vi "Sort Fcurve segment metadata.vi"(0 "reference in":refnum<class "metadata.lvclass">, 5 "error in (no error)":errorcluster) -> (14 "reference out":refnum<class "metadata.lvclass">, 19 "error out":errorcluster)   [LabVIEW 2019, in "metadata.lvclass"]
uses:
  metadata.lvclass
  Fcurve segment.ctl
  Segment type--combobox.ctl
panel:
  out "Array 3":string[][](array[string])
  out "Array":dbl[][](array[numeric])
  out "Array 2":string[][](array[string])
  out "Fcurve segment":T1[](array[typedef])
  out "Fcurve segments":i32[][](array[numeric])
  out "number_segments":i32
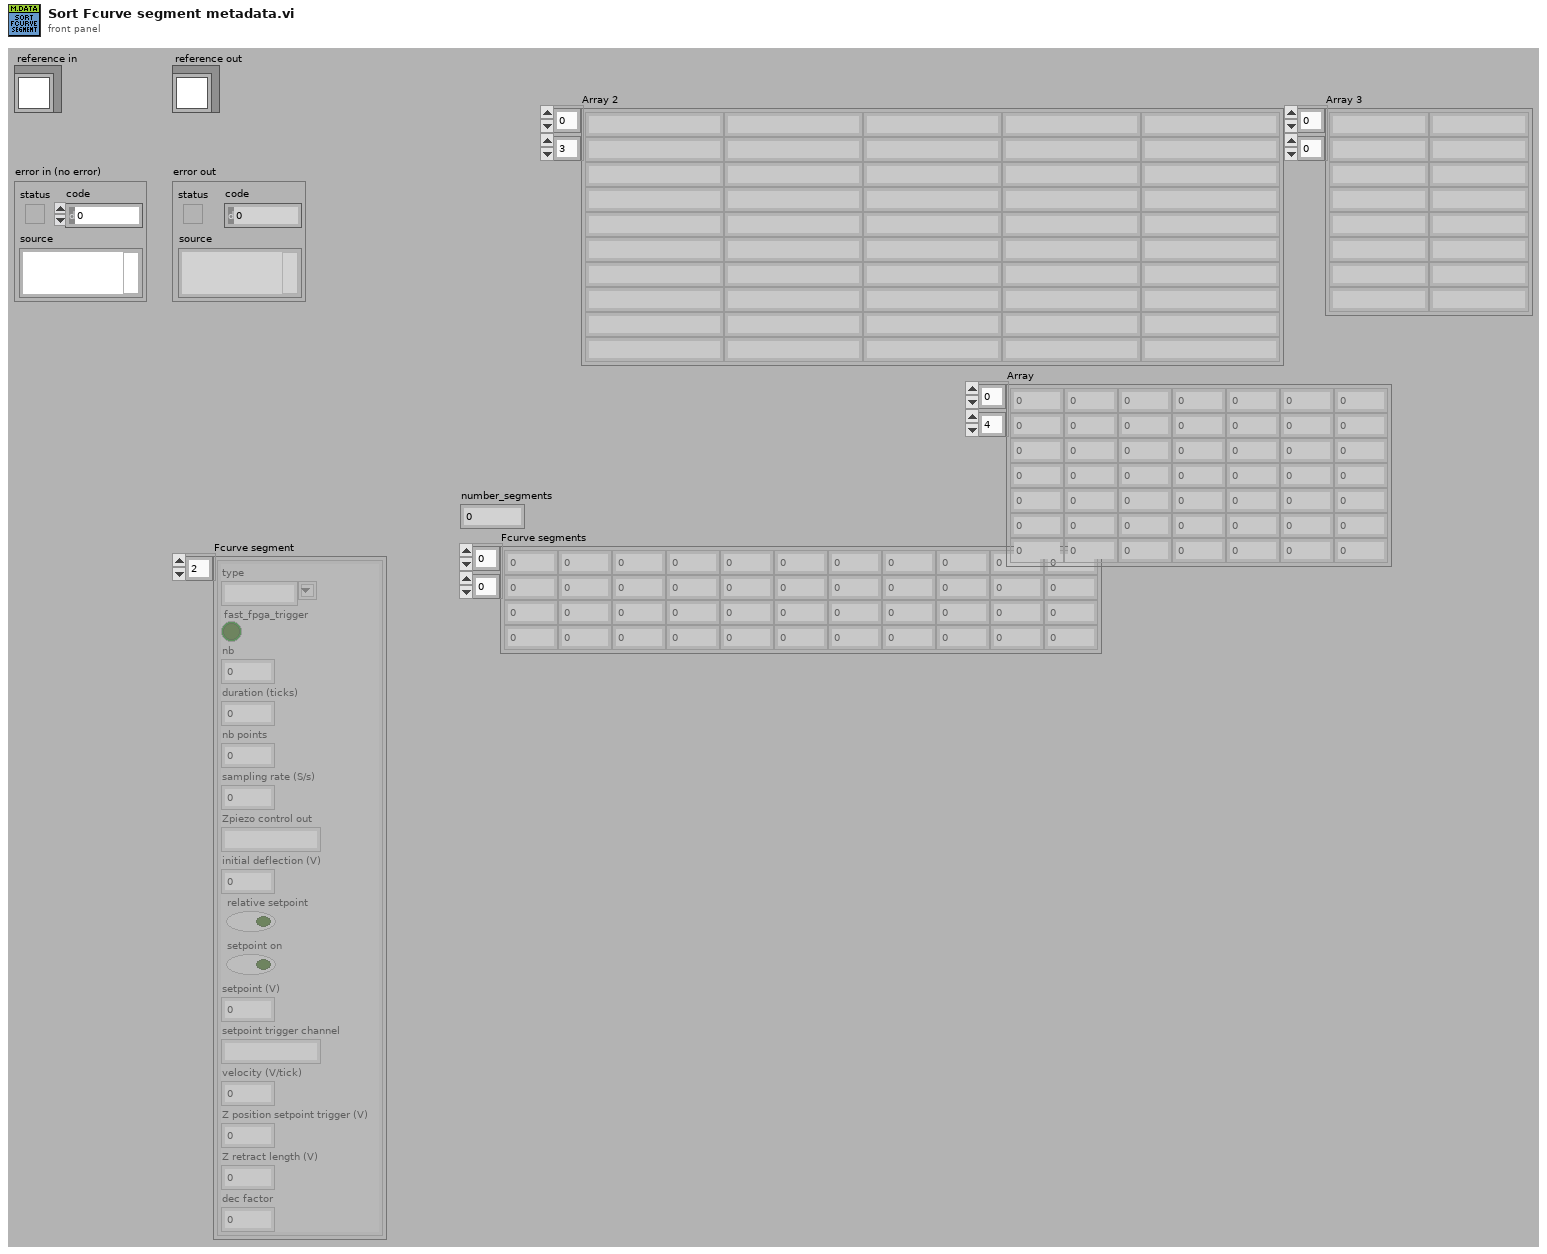
[diagram p1: front panel]
types:
  T1 = typedef "metadata.lvclass/Fcurve segment.ctl" = cluster{"type":T2, "fast_fpga_trigger":bool, "nb":u8, "duration (ticks)":i64, "nb points":i32, "sampling rate (S/s)":u32, "Zpiezo control out":string, "initial deflection (V)":dbl, "relative setpoint":bool, "setpoint on":bool, "setpoint (V)":dbl, "setpoint trigger channel":string, "velocity (V/tick)":dbl, "Z position setpoint trigger (V)":dbl, "Z retract length (V)":dbl, "dec factor":u32}
  T2 = typedef "metadata.lvclass/Segment type--combobox.ctl" = string
  T3 = typedef "metadata.lvclass/ObjectAttributesRef.ctl" = refnum<data-value>
  T4 = typedef "metadata.lvclass/ObjectAttributes.ctl" = cluster{"MyAttribute":dbl, "System Control":T5, "file info":T6, "Sample info":T7, "Cantilever info":T8, "XYZ piezos":T9, "Mapping":T10, "Fcurve segment":T1[], "Fast fpga segment":T11, "Chirp":T12, "precision (6)":i16, "width (-)":i16, "Metadata":T13, "config filepath":path, "Section names []":string[], "Property names []":string[], "nb elements":u16}
  T5 = typedef "metadata.lvclass/System control parameters.ctl" = cluster{"FPGA SW version":string, "TDMS file version":string, "Instrument":string, "Instrument model":string, "Instrument scanner":string, "Instrument clockrate (Mhz)":string, "Instrument tick time (us)":string}
  T6 = typedef "metadata.lvclass/File info parameters.ctl" = cluster{"Time Stamp":timestamp, "Filename":string, "Filepath":path, "User":string, "Experiment_name":string, "Curve_id":string, "number_segments":u8, "number_consecutive_scans":u32}
  T7 = typedef "metadata.lvclass/Sample info parameters.ctl" = cluster{"Sample name":string, "Sample species":string}
  T8 = typedef "metadata.lvclass/Cantilever info parameters.ctl" = cluster{"spring constant calib method":string, "invOLS calib method":string, "thermal calib deflection channel":string, "model":string, "shape":string, "tip geometry":string, "Laser sum (V)":dbl, "Laser power (mA)":dbl, "invOLS_(nm/V)":dbl, "spring constant nominal (N/m)":dbl, "spring constant calib (N/m)":dbl, "resosnance frequency air calib (Hz)":dbl, "resosnance frequency calib (Hz)":dbl, "quality factor":dbl, "Acoefficident_GCI_(nN.s^1.3/m)":dbl, "half angle (deg)":dbl, "tip radius (m)":dbl, "tip height (m)":dbl, "system mount angle (deg)":dbl}
  T9 = typedef "metadata.lvclass/XYZ piezos parameters.ctl" = cluster{"X stage piezo sensitivity (nm/V)":dbl, "X stage piezo gain":dbl, "X velocity (V/tick)":dbl, "X closed loop":bool, "Y stage piezo sensitivity (nm/V)":dbl, "Y stage piezo gain":dbl, "Y velocity (V/tick)":dbl, "Y closed loop":bool, "Z stage piezo sensitivity (nm/V)":dbl, "Z stage piezo gain":dbl, "Z closed loop":bool, "X position (V)":dbl, "Y position (V)":dbl}
  T10 = typedef "metadata.lvclass/Mapping parameters.ctl" = cluster{"Mapping":bool, "index":u16, "position row":u16, "position column":u16, "next position row":i16, "next position column":i16, "X initial position (V)":dbl, "Y initial position (V)":dbl, "X step size (V)":dbl, "Y step size (V)":dbl}
  T11 = typedef "metadata.lvclass/fast fpga segment parameters.ctl" = cluster{"Fast start time trigger":timestamp, "nb_points":u32, "sampling_rate_(S/s)":u32, "duration_(ticks)":u32}
  T12 = typedef "metadata.lvclass/Chirp added parameters.ctl" = cluster{"f start (Hz)":dbl, "f end (Hz)":dbl, "Sweep type":string}
  T13 = typedef "metadata.lvclass/Metadata output --cluster.ctl" = cluster{"Property Names":string[], "Property Values":variant[]}
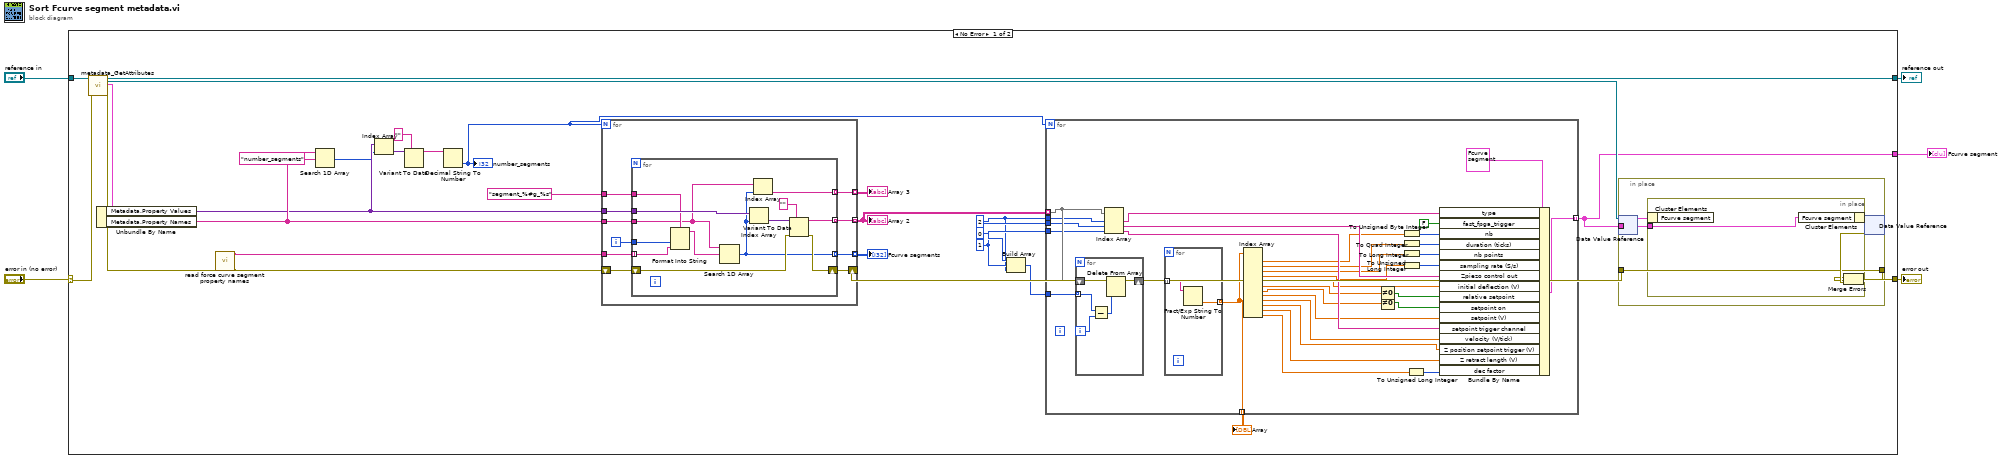
[diagram p0: block diagram]
diagram:
  n1 = case shown="No Error" "error in (no error)" {
    selector: "error in (no error)" -> [w31 w104]
    tunnel: [w35 w104] -> w4
    tunnel: [w30 w103] -> w2
    tunnel: "reference in" -> [w32 w103]
    tunnel: [w15 _] -> w1
    frame No Error {
      w9 = 1 ("index")
      w10 = 0 ("index")
      w8 = 2 ("index")
      n2 = call "metadata_GetAttributes.vi"("reference in"=w32, "error in (no error)"=w31) -> ("reference out"=w30:refnum<class "metadata.lvclass">, "attributes ref"=w29:T3, "attributes"=w28:T4, "error out"=w26:errorcluster)  [unwired: 14 in]
      n3 = Unbundle By Name(w28) -> ("Metadata.Property Values"=w21:variant[], "Metadata.Property Names"=w23:string[])
      n4 = call "read force curve segment property names.vi"("error in (no error)"=w26) -> ("Fcurve Seg"=w24:string[], "error out"=w25:errorcluster)  [unwired: 17 in]
      n5 = Search 1D Array(1D array=w23, element="number_segments") -> (index of element=w20:i32)  [unwired: 1 in]
      n6 = Index Array(array=w21, index=w20) -> (element=w18:variant)
      n7 = Variant To Data(type="", Variant=w18) -> (data=w17:string)  [unwired: 1 in, 1 out]
      n8 = Decimal String To Number(string=w17) -> (number=w14:i32)  [unwired: 2 in, 1 out]
      "number_segments" <- w14
      n9 = for {
        N: w14 -> [_]
        tunnel: w24 -> [w84]
        tunnel: [w81] -> w13 mode=indexing
        shift-right: [w78] -> w27
        shift-left: w25 -> [w79]
        tunnel: w23 -> [w83]
        tunnel: w21 -> [w82]
        tunnel: [w80] -> w12 mode=indexing
        tunnel: "segment_%#g_%s" ("format string") -> [w77]
        tunnel: [w75] -> w6 mode=indexing
        i -> [w76]
        n10 = for {
          tunnel: w84 -> [w89] mode=indexing
          tunnel: w83 -> [w87]
          tunnel: w82 -> [w97]
          tunnel: [w86] -> w81 mode=indexing
          tunnel: [w95] -> w80 mode=indexing
          shift-right: [w93] -> w78
          shift-left: w79 -> [w94]
          tunnel: w77 -> [w91]
          tunnel: w76 -> [w90]
          tunnel: [w85] -> w75 mode=indexing
          n11 = Format Into String(format string=w91, w90, w89) -> (resulting string=w88:string)  [unwired: 2 in, 1 out]
          n12 = Search 1D Array(1D array=w87, element=w88) -> (index of element=w86:i32)  [unwired: 1 in]
          n13 = Index Array(array=w97, index=w86) -> (element=w96:variant)
          n14 = Index Array(array=w87, index=w86) -> (element=w85:string)
          n15 = Variant To Data(error in=w94, type="", Variant=w96) -> (data=w95:string, error out=w93:errorcluster)
        }
      }
      "Fcurve segments" <- w13
      "Array 2" <- w12
      "Array 3" <- w6
      n16 = Build Array(w10, w9, w8) -> (w11:i32[])
      n17 = for {
        N: w14 -> [_]
        tunnel: [w67] -> w15 mode=indexing
        tunnel: w12 -> [w62] mode=indexing
        tunnel: w9 -> [w61]
        tunnel: w10 -> [w60]
        tunnel: w8 -> [w59]
        tunnel: w11 -> [w58]
        tunnel: [w56] -> w7 mode=indexing
        n18 = for {
          shift-right: [w73] -> w57
          shift-left: w62 -> [w74]
          tunnel: w58 -> [w72] mode=indexing
          i -> [w71]
          n19 = Subtract(x=w72, y=w71) -> (x-y=w70:i32)
          n20 = Delete From Array(array=w74, index=w70) -> (array with subset deleted=w73:string[])  [unwired: 1 in, 1 out]
        }
        n21 = Index Array(array=w62, index #1=w59, index #2=w60, index #3=w61) -> (element #1=w65:string, element #2=w64:string, element #3=w63:string)
        n22 = for {
          tunnel: w57 -> [w69] mode=indexing
          tunnel: [w68] -> w56 mode=indexing
          n23 = Fract/Exp String To Number(string=w69) -> (number=w68:dbl)  [unwired: 3 in, 1 out]
        }
        n24 = Index Array(array=w56) -> (element #1=w54:dbl, element #2=w53:dbl, element #3=w50:dbl, element #4=w48:dbl, element #5=w47:dbl, element #6=w46:dbl, element #7=w45:dbl, element #8=w42:dbl, element #9=w41:dbl, element #10=w40:dbl, element #11=w39:dbl, element #12=w37:dbl)  [unwired: 12 in]
        n25 = Not Equal To 0?(x=w46) -> (x != 0?=w44:bool)
        n26 = Not Equal To 0?(x=w45) -> (x != 0?=w43:bool)
        n27 = To Unsigned Byte Integer(number=w54) -> (unsigned 8bit integer=w55:u8)
        n28 = To Quad Integer(1:w53) -> (0:w52:i64)
        n29 = To Long Integer(number=w50) -> (32bit integer=w51:i32)
        n30 = To Unsigned Long Integer(number=w48) -> (unsigned 32bit integer=w49:u32)
        n31 = To Unsigned Long Integer(number=w37) -> (unsigned 32bit integer=w38:u32)
        n32 = Bundle By Name(cluster=T1 {"type"="App", "fast_fpga_trigger"=FALSE, "nb"=0, "duration (ticks)"=0, "nb points"=0, "sampling rate (S/s)"=0, "Zpiezo control out"="", "initial deflection (V)"=0.0, "relative setpoint"=FALSE, "setpoint on"=FALSE, "setpoint (V)"=0.0, "setpoint trigger channel"="", "velocity (V/tick)"=0.0, "Z position setpoint trigger (V)"=0.0, "Z retract length (V)"=0.0, "dec factor"=0} ("Fcurve segment"), "type"=w65, "fast_fpga_trigger"=FALSE, "nb"=w55, "duration (ticks)"=w52, "nb points"=w51, "sampling rate (S/s)"=w49, "Zpiezo control out"=w64, "initial deflection (V)"=w47, "relative setpoint"=w44, "setpoint on"=w43, "setpoint (V)"=w42, "setpoint trigger channel"=w63, "velocity (V/tick)"=w41, "Z position setpoint trigger (V)"=w40, "Z retract length (V)"=w39, "dec factor"=w38) -> (w67:T1)
      }
      "Array" <- w7
      n33 = in-place {
        in-place-border: w27 -> [w99]
        in-place-border: [w99] -> w33
        in-place-border: w15 -> [w98]
        n34 = in-place-dvr #1(w29) -> (w100:T4)  [unwired: 1 out]
        n35 = in-place {
          in-place-border: w98 -> [w102]
          n36 = in-place-cluster #2(w100) -> ()  [unwired: 1 out]
          n37 = in-place-cluster #2("Fcurve segment"=w102) -> (w101:T4)
        }
        n38 = in-place-dvr #1(w101) -> (w34:errorcluster)  [unwired: 1 out]
      }
      n39 = Merge Errors(w33, w34) -> (w35:errorcluster)
    }
    frame Error {
    }
  }
  "error out" <- w4
  "reference out" <- w2
  "Fcurve segment" <- w1
